vi "Obtain Request Events.vi"(8 "error in":errorcluster, 10 "Create New? (F)":bool) -> (0 "error out":errorcluster, 2 "FunctionGenerator Request Events":T1)   [LabVIEW 2019, in "FunctionGenerator.lvlib"]
doc: "This VI Obtains/Creates the Requests events that will be used for other modules to communicate with the module that owns this VI. These Requests events will be accessed only via Public API methods for this module.\n\n<b>NOTE</b>: The contents of this VI are automatically generated and modified by the <b>Tools > DQMH Consortium > DQMH</b> utilities. Consider using those utilities instead of making your own modifications to this VI.\n_____\nBased on DQMH Dev Tools: Project Template 7.1.0.1503."
uses:
  FunctionGenerator.lvlib
  Request Events--cluster.ctl
  Stop Argument--cluster.ctl
  Show Panel Argument--cluster.ctl
  Hide Panel Argument--cluster.ctl
  Get Module Execution Status Argument--cluster.ctl
  Show Diagram Argument--cluster.ctl
  Set Amplitude Argument--cluster.ctl
  Set Offset Argument--cluster.ctl
  Set Frecuency Argument--cluster.ctl
  Set Signal Type Argument--cluster.ctl
  Get Waveform Argument--cluster.ctl
  Get Waveform (Reply Payload)--cluster.ctl
  Wake UP Continuous HL Argument--cluster.ctl
  Start Continuous Acquisition Argument--cluster.ctl
  Stop Continuous Generation Argument--cluster.ctl
panel:
  # "NOTE: The contents of this VI are automatically generated and modified by the Tools > DQMH Consortium > DQMH utilities. Consider using those utilities instead of making your own modifications to this VI."
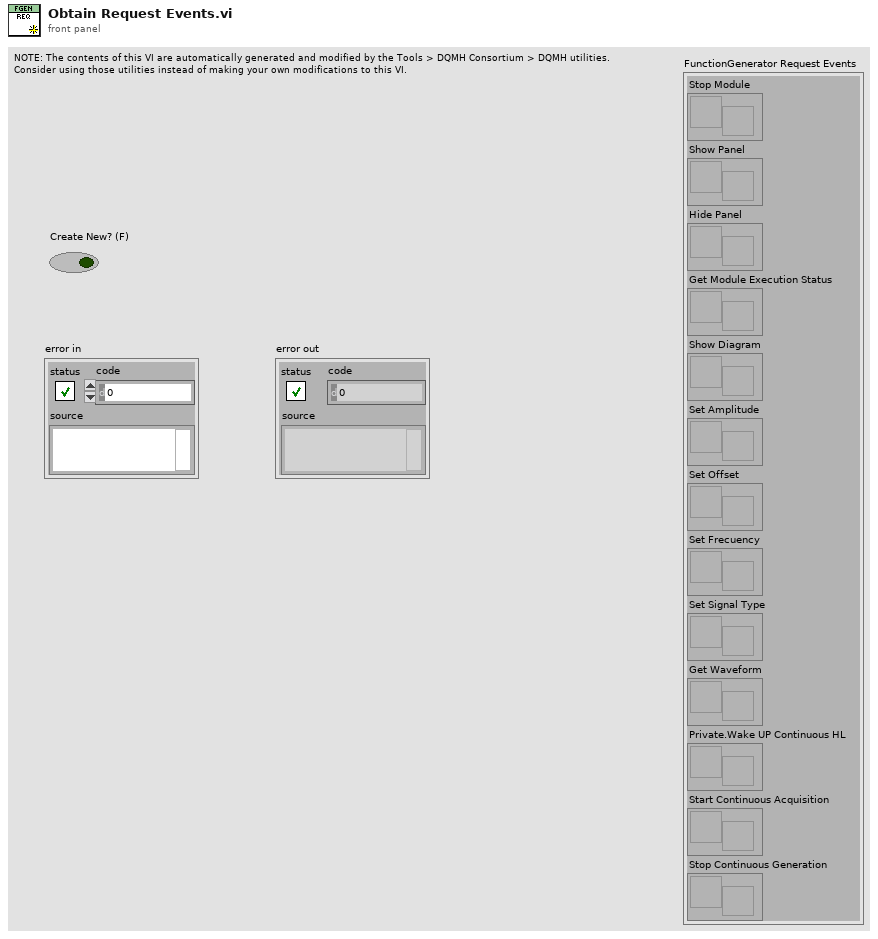
[diagram p1: front panel]
types:
  T1 = typedef "FunctionGenerator.lvlib/Request Events--cluster.ctl" = cluster{"Stop Module":refnum<user-event>, "Show Panel":refnum<user-event>, "Hide Panel":refnum<user-event>, "Get Module Execution Status":refnum<user-event>, "Show Diagram":refnum<user-event>, "Set Amplitude":refnum<user-event>, "Set Offset":refnum<user-event>, "Set Frecuency":refnum<user-event>, "Set Signal Type":refnum<user-event>, "Get Waveform":refnum<user-event>, "Private.Wake UP Continuous HL":refnum<user-event>, "Start Continuous Acquisition":refnum<user-event>, "Stop Continuous Generation":refnum<user-event>}
  T2 = typedef "FunctionGenerator.lvlib/Stop Continuous Generation Argument--cluster.ctl" = cluster{"Boolean":bool}
  T3 = typedef "FunctionGenerator.lvlib/Start Continuous Acquisition Argument--cluster.ctl" = cluster{"Boolean":bool}
  T4 = typedef "FunctionGenerator.lvlib/Wake UP Continuous HL Argument--cluster.ctl" = cluster{"Amplitude":dbl, "Frecuency":dbl, "Offset":dbl, "signal type":enum16{"Sine Wave", "Triangle Wave", "Square Wave", "Sawtooth Wave"}}
  T5 = typedef "FunctionGenerator.lvlib/Get Waveform Argument--cluster.ctl" = cluster{"Wait Notifier":refnum<notifier>, "wait for reply":bool}
  T6 = typedef "FunctionGenerator.lvlib/Set Signal Type Argument--cluster.ctl" = cluster{"signal type":enum16{"Sine Wave", "Triangle Wave", "Square Wave", "Sawtooth Wave"}}
  T7 = typedef "FunctionGenerator.lvlib/Set Frecuency Argument--cluster.ctl" = cluster{"Frecuency":dbl}
  T8 = typedef "FunctionGenerator.lvlib/Set Offset Argument--cluster.ctl" = cluster{"Offset":dbl}
  T9 = typedef "FunctionGenerator.lvlib/Set Amplitude Argument--cluster.ctl" = cluster{"Amplitude":dbl}
  T10 = typedef "FunctionGenerator.lvlib/Hide Panel Argument--cluster.ctl" = cluster{"Hide Panel?":bool}
  T11 = typedef "FunctionGenerator.lvlib/Show Panel Argument--cluster.ctl" = cluster{"Show Panel?":bool}
  T12 = typedef "FunctionGenerator.lvlib/Show Diagram Argument--cluster.ctl" = cluster{"Debug?":bool}
  T13 = typedef "FunctionGenerator.lvlib/Get Module Execution Status Argument--cluster.ctl" = cluster{"Running?":bool}
  T14 = typedef "FunctionGenerator.lvlib/Stop Argument--cluster.ctl" = cluster{"Origin":string, "Exit via Stop Module Req?":bool, "Wait for Module to stop?":bool}
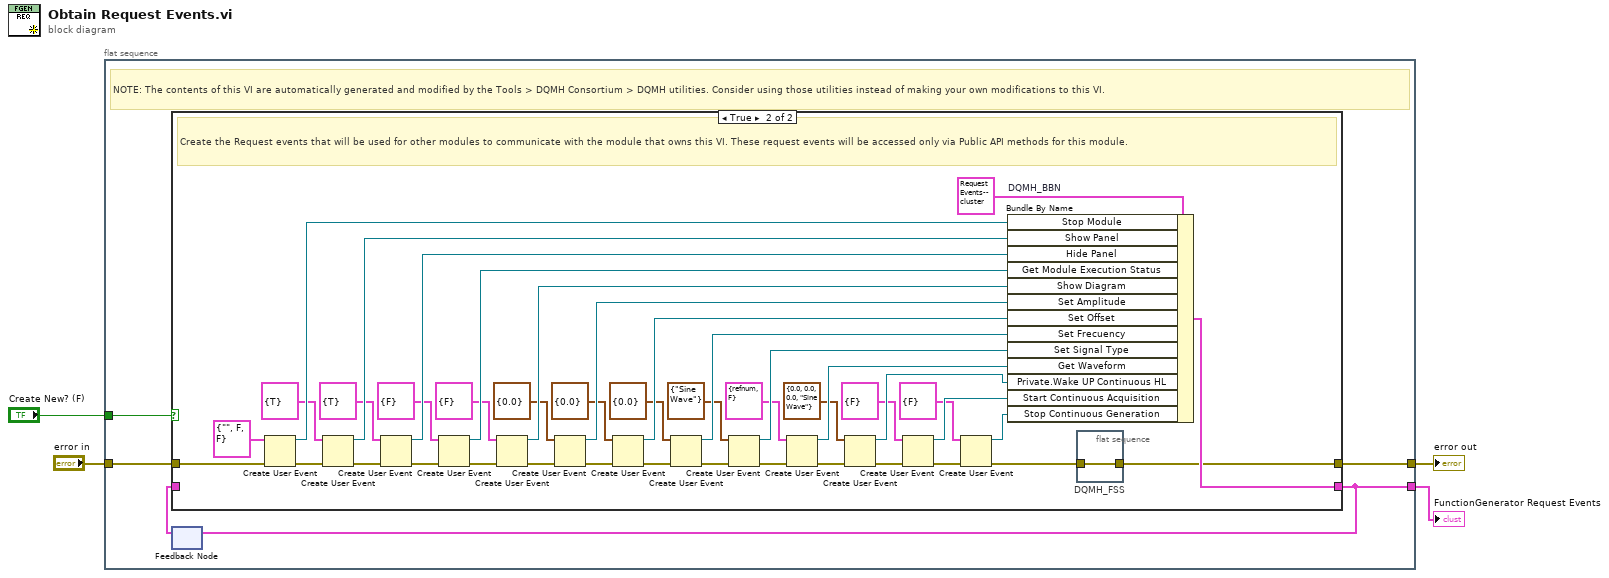
[diagram p0: block diagram]
diagram:
  n1 = flat-sequence {
    tunnel: [w9] -> w4
    tunnel: "error in" -> [w8]
    tunnel: [w6] -> w2
    tunnel: "Create New? (F)" -> [w5]
    frame #0 {
      # "NOTE: The contents of this VI are automatically generated and modified by the Tools > DQMH Consortium > DQMH utilities. Consider using those utilities instead of making your own modifications to this VI."
      n2 = feedback #1() -> (w7:T1)  [unwired: 1 in]
      n3 = case shown="True" w5 {
        tunnel: [w10 w44] -> w9
        tunnel: w8 -> [w10 w54]
        tunnel: [w11 w51] -> w6
        tunnel: w7 -> [w11 _]
        frame False {
          # "Obtain the Request events that were created in a previous call to this VI."
        }
        frame True {
          # "Create the Request events that will be used for other modules to communicate with the module that owns this VI. These request events will be accessed only via Public API methods for this module."
          n4 = Create User Event(user event datatype=T14 {"Origin"="", "Exit via Stop Module Req?"=FALSE, "Wait for Module to stop?"=FALSE} ("Stop Argument"), error in=w54) -> (user event=w52:refnum<user-event>, error out=w49:errorcluster)
          n5 = Create User Event(user event datatype=T11 {"Show Panel?"=TRUE} ("Show Panel Argument"), error in=w49) -> (user event=w48:refnum<user-event>, error out=w47:errorcluster)
          n6 = Create User Event(user event datatype=T10 {"Hide Panel?"=TRUE} ("Hide Panel Argument"), error in=w47) -> (user event=w46:refnum<user-event>, error out=w45:errorcluster)
          n7 = Create User Event(user event datatype=T13 {"Running?"=FALSE} ("Get Module Execution Status Argument"), error in=w45) -> (user event=w42:refnum<user-event>, error out=w43:errorcluster)
          n8 = Create User Event(user event datatype=T12 {"Debug?"=FALSE} ("Show Diagram Argument"), error in=w43) -> (user event=w39:refnum<user-event>, error out=w40:errorcluster)
          n9 = Create User Event(user event datatype=T9 {"Amplitude"=0.0} ("Set Amplitude Argument"), error in=w40) -> (user event=w34:refnum<user-event>, error out=w35:errorcluster)
          n10 = Create User Event(user event datatype=T8 {"Offset"=0.0} ("Set Offset Argument"), error in=w35) -> (user event=w31:refnum<user-event>, error out=w32:errorcluster)
          n11 = Create User Event(user event datatype=T7 {"Frecuency"=0.0} ("Set Frecuency Argument"), error in=w32) -> (user event=w28:refnum<user-event>, error out=w29:errorcluster)
          n12 = Create User Event(user event datatype=T6 {"signal type"=enum."Sine Wave"} ("Set Signal Type Argument"), error in=w29) -> (user event=w25:refnum<user-event>, error out=w26:errorcluster)
          n13 = Create User Event(user event datatype=T5 {"Wait Notifier"=refnum, "wait for reply"=FALSE} ("Get Waveform Argument"), error in=w26) -> (user event=w22:refnum<user-event>, error out=w23:errorcluster)
          n14 = Create User Event(user event datatype=T4 {"Amplitude"=0.0, "Frecuency"=0.0, "Offset"=0.0, "signal type"=enum."Sine Wave"} ("Wake UP Continuous HL Argument"), error in=w23) -> (user event=w19:refnum<user-event>, error out=w20:errorcluster)
          n15 = Create User Event(user event datatype=T3 {"Boolean"=FALSE} ("Start Continuous Acquisition Argument"), error in=w20) -> (user event=w16:refnum<user-event>, error out=w17:errorcluster)
          n16 = Create User Event(user event datatype=T2 {"Boolean"=FALSE} ("Stop Continuous Generation Argument"), error in=w17) -> (user event=w13:refnum<user-event>, error out=w14:errorcluster)
          n17 = Bundle By Name "DQMH_BBN"(cluster=T1 {"Stop Module"=refnum, "Show Panel"=refnum, "Hide Panel"=refnum, "Get Module Execution Status"=refnum, "Show Diagram"=refnum, "Set Amplitude"=refnum, "Set Offset"=refnum, "Set Frecuency"=refnum, "Set Signal Type"=refnum, "Get Waveform"=refnum, "Private.Wake UP Continuous HL"=refnum, "Start Continuous Acquisition"=refnum, "Stop Continuous Generation"=refnum} ("output cluster"), "Stop Module"=w52, "Show Panel"=w48, "Hide Panel"=w46, "Get Module Execution Status"=w42, "Show Diagram"=w39, "Set Amplitude"=w34, "Set Offset"=w31, "Set Frecuency"=w28, "Set Signal Type"=w25, "Get Waveform"=w22, "Private.Wake UP Continuous HL"=w19, "Start Continuous Acquisition"=w16, "Stop Continuous Generation"=w13) -> (w51:T1)
          n18 = flat-sequence "DQMH_FSS" {
            tunnel: w14 -> [w55]
            tunnel: [w55] -> w44
            frame #0 {
            }
          }
        }
      }
      n19 = feedback-in #1(w6) -> ()
    }
  }
  "FunctionGenerator Request Events" <- w2
  "error out" <- w4
